vi "Hardware Test - GUI.vi"() -> ()   [LabVIEW 2020]
uses:
  <vilib>/Platform/TimedLoop/XDataNode/timing_clust.ctl
  <vilib>/Platform/TimedLoop/XDataNode/nitl_modes.ctl
  <vilib>/Platform/TimedLoop/XDataNode/wakeup.ctl
  <vilib>/Instr/_visa.llb/VISA Configure Serial Port (Instr).vi
  <vilib>/platform/TimedLoop/XDataNode/XDataNode.xnode
  <vilib>/Platform/TimedLoop/XDataNode/XDNodeRunTimeDep.lvlib
panel:
  out "return count":u32
  in  "stop":bool
  out "Blue Workpiece":bool
  out "Green Workpiece":bool
  out "Red Workpiece":bool
  out "Push Button":bool
  out "Proximity":bool
  out "IR Slider 3":bool
  out "IR Slider 2":bool
  out "IR Slider 1":bool
  out "IR Conveyor":bool
  out "IR Stack":bool
  in  "VISA resource name":refnum<visa-resource-name>
  in  "write buffer":string
  out "read buffer":string
  in  "byte count":u32
  in  "Menu":u16(ring) items=["Idle", "Infrared Sensors", "Proximity Sensor & Button", "Servo Linear", "Servo Slider", "Conveyor", "LED Indicator", "Color Sensor"]
  # "INFRARED SENSORS"
  # "TRAINER ARDUINO\nMPS SORTING STATION"
  # "PROXIMITY SENSOR & PUSH BUTTON"
  # "Mechatronics Engineering 2nd Generation\n  Vocational High School 2 Bojonegoro\n2021"
  # "COLOR SENSOR DETECTION"
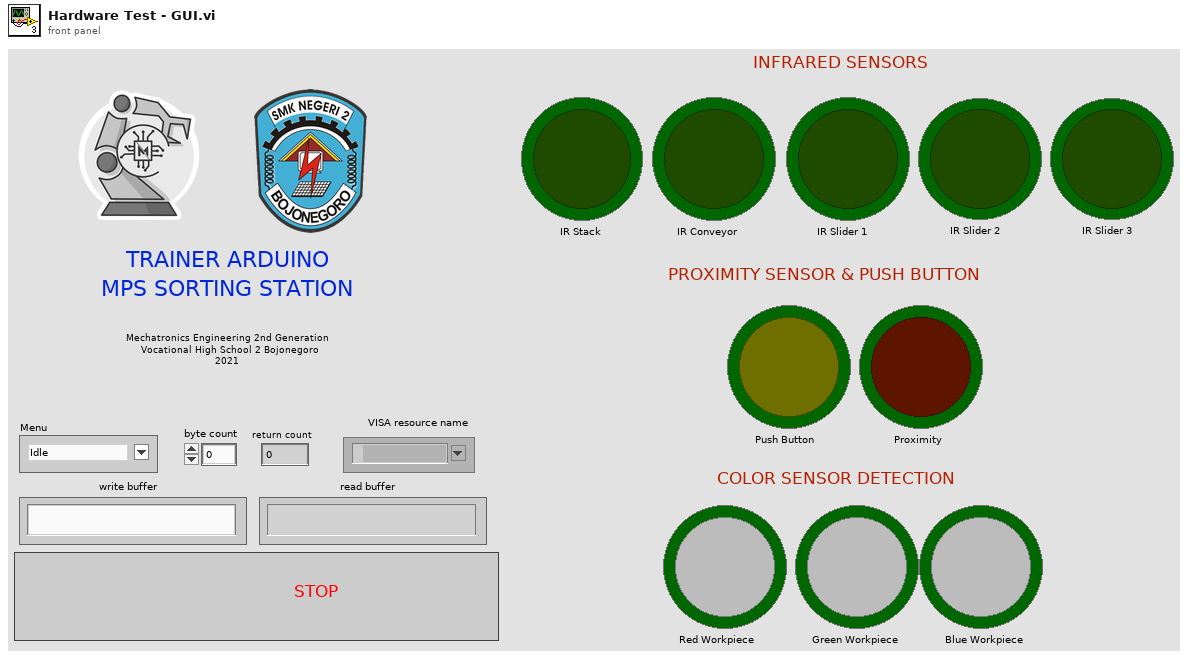
[diagram p1: front panel]
types:
  T1 = typedef "XDNodeRunTimeDep.lvlib/timing_clust.ctl" = cluster{"Expected End [f-1]":u64, "Actual End [f-1]":u64, "Finished Late? [f-1]":bool, "Expected End [i-1]":u64, "Actual End [i-1]":u64, "Finished Late? [i-1]":bool, "Expected Start [i]":u64, "Actual Start [i]":u64, "Expected Start [f]":u64, "Actual Start [f]":u64, "Source Name":string, "Structure Name":string, "Period":i64, "Deadline":i64, "Offset":i64, "Start":i64, "Priority":i32, "Timeout":i32, "Mode":T2, "Wakeup Reason":T3, "Error":errorcluster, "Source Type":string, "Secondary Source Type":string, "Global End Time":u64, "Global Start Time":u64, "Frame Duration":u64, "Iteration Duration":u64, "Assigned CPU":i32, "I/O Scan Engine Mode":u32}
  T2 = typedef "XDNodeRunTimeDep.lvlib/nitl_modes.ctl" = enum32{"No Change", "Process missed periods, maintain original phase", "Discard missed periods, maintain original phase", "Process missed periods, ignore original phase", "Discard missed periods, ignore original phase"}
  T3 = typedef "XDNodeRunTimeDep.lvlib/wakeup.ctl" = enum32{"Normal", "Aborted", "Asynchronous wakeup", "Timing source error", "Timed loop error", "Timeout"}
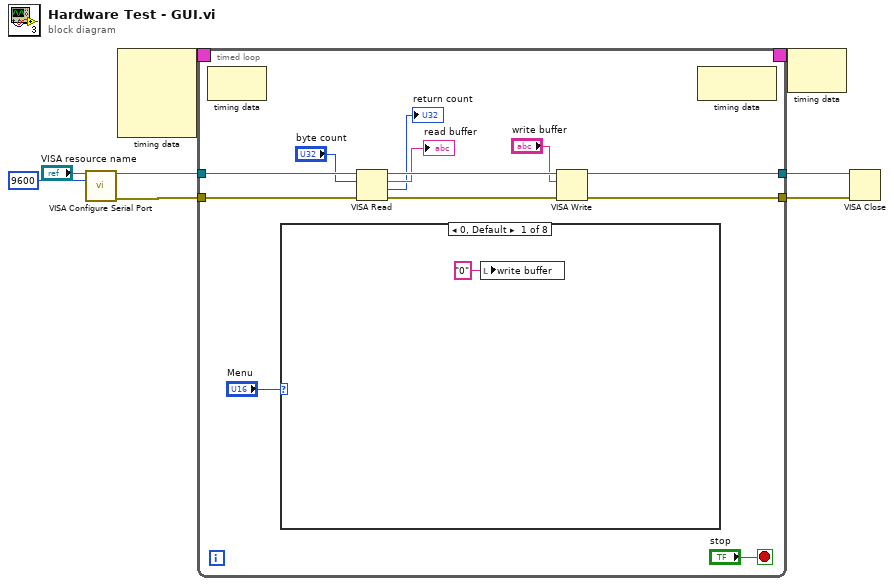
[diagram p0: block diagram]
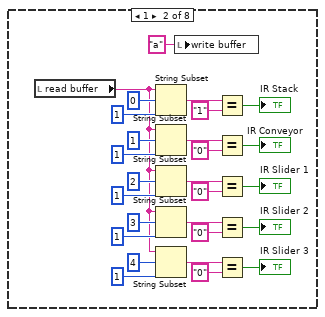
[diagram p2: hidden frame]
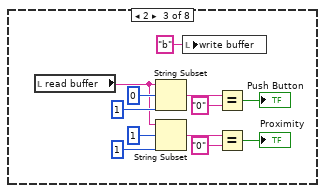
[diagram p3: hidden frame]
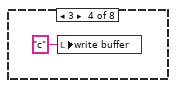
[diagram p4: hidden frame]
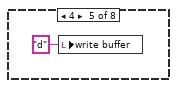
[diagram p5: hidden frame]
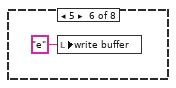
[diagram p6: hidden frame]
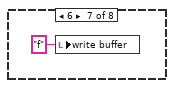
[diagram p7: hidden frame]
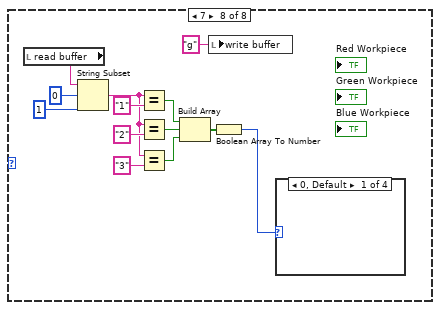
[diagram p8: hidden frame]
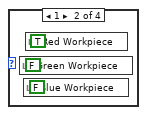
[diagram p9: hidden frame]
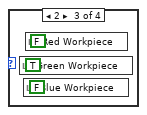
[diagram p10: hidden frame]
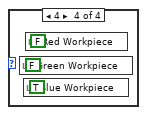
[diagram p11: hidden frame]
diagram:
  n1 = call-poly "VISA Configure Serial Port"("VISA resource name"="VISA resource name", "baud rate (9600)"=u32 9600) -> ("VISA resource name out"=w6:refnum<visa-resource-name>, "error out"=w5:errorcluster)  [unwired: 12 in]
  n2 = node-c288() -> (w8:T1)  [unwired: 4 in]
  n3 = timed-loop {
    timing: w8 -> [_]
    timing-out: [_] -> w7
    tunnel: w6 -> [w20]
    tunnel: w5 -> [w19]
    tunnel: [w16] -> w4
    tunnel: [w15] -> w3
    stop <- "stop" stop-if-true
    n4 = node-c288() -> ()  [unwired: 1 in, 1 out]
    n5 = case shown="0, Default" "Menu" {
      frame 0, Default {
        n6 = local write "write buffer"("0" ("write buffer")) -> ()
      }
      frame 1 {
        n7 = local read "read buffer"() -> (w38:string)
        n8 = String Subset(string=w38, offset (0)=0, length (rest)=1 ("length (rest)")) -> (substring=w37:string)
        n9 = String Subset(string=w38, offset (0)=1, length (rest)=1 ("length (rest)")) -> (substring=w28:string)
        n10 = String Subset(string=w38, offset (0)=2, length (rest)=1 ("length (rest)")) -> (substring=w29:string)
        n11 = String Subset(string=w38, offset (0)=3, length (rest)=1 ("length (rest)")) -> (substring=w30:string)
        n12 = String Subset(string=w38, offset (0)=4, length (rest)=1 ("length (rest)")) -> (substring=w31:string)
        n13 = local write "write buffer"("a" ("write buffer")) -> ()
        n14 = Equal?(x=w37, y="1") -> (x = y?=→"IR Stack":bool)
        n15 = Equal?(x=w28, y="0") -> (x = y?=→"IR Conveyor":bool)
        n16 = Equal?(x=w29, y="0") -> (x = y?=→"IR Slider 1":bool)
        n17 = Equal?(x=w30, y="0") -> (x = y?=→"IR Slider 2":bool)
        n18 = Equal?(x=w31, y="0") -> (x = y?=→"IR Slider 3":bool)
      }
      frame 2 {
        n19 = local read "read buffer"() -> (w55:string)
        n20 = String Subset(string=w55, offset (0)=0, length (rest)=1 ("length (rest)")) -> (substring=w54:string)
        n21 = String Subset(string=w55, offset (0)=1, length (rest)=1 ("length (rest)")) -> (substring=w51:string)
        n22 = local write "write buffer"("b" ("write buffer")) -> ()
        n23 = Equal?(x=w54, y="0") -> (x = y?=→"Push Button":bool)
        n24 = Equal?(x=w51, y="0") -> (x = y?=→"Proximity":bool)
      }
      frame 3 {
        n25 = local write "write buffer"("c" ("write buffer")) -> ()
      }
      frame 4 {
        n26 = local write "write buffer"("d" ("write buffer")) -> ()
      }
      frame 5 {
        n27 = local write "write buffer"("e" ("write buffer")) -> ()
      }
      frame 6 {
        n28 = local write "write buffer"("f" ("write buffer")) -> ()
      }
      frame 7 {
        n29 = local read "read buffer"() -> (w74:string)
        n30 = String Subset(string=w74, offset (0)=0, length (rest)=1 ("length (rest)")) -> (substring=w70:string)
        n31 = Equal?(x=w70, y="1") -> (x = y?=w67:bool)
        n32 = Equal?(x=w70, y="2") -> (x = y?=w68:bool)
        n33 = Equal?(x=w70, y="3") -> (x = y?=w69:bool)
        n34 = Build Array(w67, w68, w69) -> (w66:bool[])
        n35 = local write "write buffer"("g" ("write buffer")) -> ()
        n36 = Boolean Array To Number(Boolean array=w66) -> (number=w65:u32)
        n37 = case shown="0, Default" w65 {
          frame 0, Default {
          }
          frame 1 {
            n38 = local write "Green Workpiece"(FALSE ("Green")) -> ()
            n39 = local write "Blue Workpiece"(FALSE ("Blue")) -> ()
            n40 = local write "Red Workpiece"(TRUE ("Red")) -> ()
          }
          frame 2 {
            n41 = local write "Green Workpiece"(TRUE ("Green")) -> ()
            n42 = local write "Blue Workpiece"(FALSE ("Blue")) -> ()
            n43 = local write "Red Workpiece"(FALSE ("Red")) -> ()
          }
          frame 4 {
            n44 = local write "Green Workpiece"(FALSE ("Green")) -> ()
            n45 = local write "Blue Workpiece"(TRUE ("Blue")) -> ()
            n46 = local write "Red Workpiece"(FALSE ("Red")) -> ()
          }
        }
      }
    }
    n47 = VISA Read(VISA resource name=w20, byte count="byte count", error in (no error)=w19) -> (VISA resource name out=w17:refnum<visa-resource-name>, read buffer=→"read buffer":string, return count=→"return count":u32, error out=w18:errorcluster)
    n48 = VISA Write(VISA resource name=w17, write buffer="write buffer", error in (no error)=w18) -> (VISA resource name out=w16:refnum<visa-resource-name>, error out=w15:errorcluster)  [unwired: 1 out]
    n49 = node-c288() -> ()  [unwired: 1 in, 1 out]
  }
  n50 = node-c288(w7) -> ()  [unwired: 1 out]
  n51 = VISA Close(VISA resource name=w4, error in (no error)=w3) -> ()  [unwired: 1 out]
